vi "sub_removeInvalidGuessFromQueue.vi"() -> ()   [LabVIEW 2018]
uses:
  guess.ctl
panel:
  out "no guesses left ?":bool
  in  "solver (in)":cluster{"solved":bool, "values":string[]}[][](array[cluster]) caption="solver array"
  in  "queues":T1
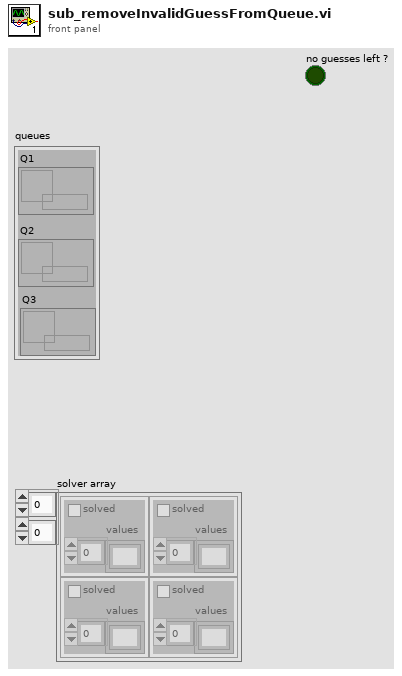
[diagram p1: front panel]
types:
  T1 = cluster{"Q1":refnum<queue>, "Q2":refnum<queue>, "Q3":refnum<queue>}
  T2 = typedef "guess.ctl" = cluster{"cell position":cluster{"row":i32, "col":i32}, "guess":string}
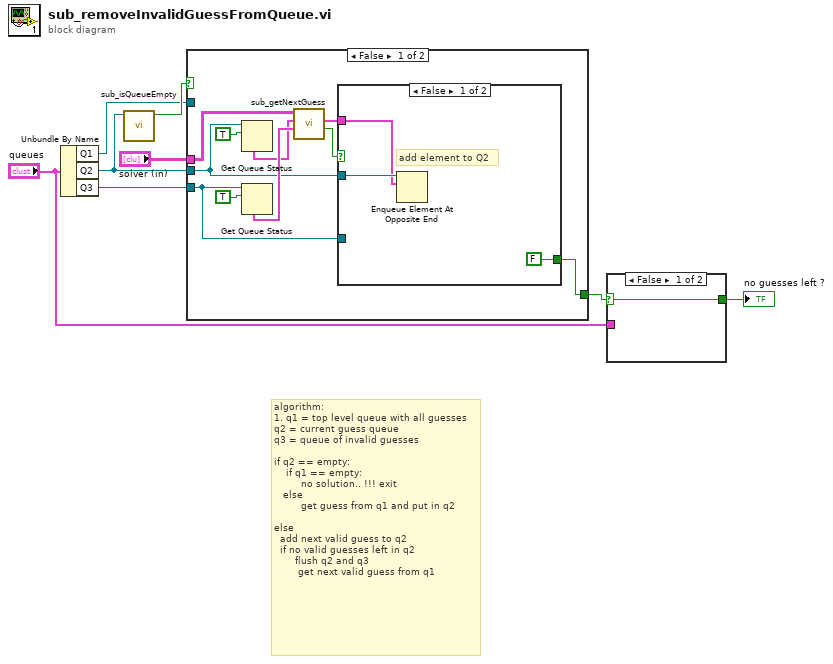
[diagram p0: block diagram]
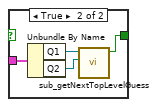
[diagram p2: hidden frame]
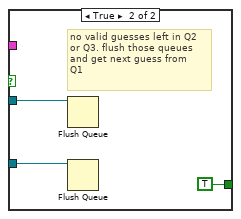
[diagram p3: hidden frame]
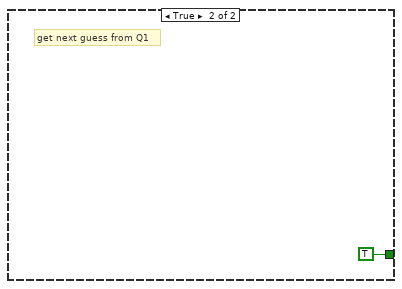
[diagram p4: hidden frame]
diagram:
  # "algorithm:\n1. q1 = top level queue with all guesses\nq2 = current guess queue\nq3 = queue of invalid guesses\n\nif q2 == empty: \n    if q1 == empty: \n         no solution.. !!! exit\n   else\n         get guess from q1 and put in q2\n\nelse\n  add next valid guess to q2\n  if no valid guesses left in q2\n       flush q2 and q3\n        get next valid guess from q1"
  n1 = Unbundle By Name("queues") -> ("Q1"=w7:refnum<queue>, "Q2"=w6:refnum<queue>, "Q3"=w5:refnum<queue>)
  n2 = call "sub_isQueueEmpty"("Q1"=w6) -> ("empty ?"=w8:bool)  [unwired: 10 in]
  n3 = case shown="False" w8 {
    tunnel: w7 -> [_ _]
    tunnel: w6 -> [w12 _]
    tunnel: w5 -> [w11 _]
    tunnel: "solver (in)" -> [w14 _]
    tunnel: [w9 TRUE] -> w3
    frame False {
      n4 = Get Queue Status(queue=w12, return elements? (F)=TRUE) -> (elements=w15:T2[])  [unwired: 1 in, 7 out]
      n5 = Get Queue Status(queue=w11, return elements? (F)=TRUE) -> (elements=w17:T2[])  [unwired: 1 in, 7 out]
      n6 = call "sub_getNextGuess.vi"("invalid guesses"=w17, "current guess queue"=w15, "solver array"=w14) -> ("no valid guess ?"=w13:bool, "next guess"=w10:T2)  [unwired: 7 in]
      n7 = case shown="False" w13 {
        tunnel: w12 -> [w21 w24]
        tunnel: w11 -> [_ w23]
        tunnel: w10 -> [w20 _]
        tunnel: [FALSE TRUE] -> w9
        frame False {
          # "add element to Q2"
          n8 = Enqueue Element At Opposite End(queue=w21, element=w20) -> ()  [unwired: 2 in, 3 out]
        }
        frame True {
          # "no valid guesses left in Q2 \nor Q3. flush those queues\nand get next guess from\nQ1"
          n9 = Flush Queue(queue=w24) -> ()  [unwired: 1 in, 3 out]
          n10 = Flush Queue(queue=w23) -> ()  [unwired: 1 in, 3 out]
        }
      }
    }
    frame True {
      # "get next guess from Q1"
    }
  }
  n11 = case shown="False" w3 {
    selector: w3 -> [w26 _]
    tunnel: "queues" -> [_ w30]
    tunnel: [w26 w27] -> w1
    frame False {
    }
    frame True {
      n12 = Unbundle By Name(w30) -> ("Q1"=w29:refnum<queue>, "Q2"=w28:refnum<queue>)
      n13 = call "sub_getNextTopLevelGuess.vi"("Q2"=w28, "Q1"=w29) -> ("q1 empty ?"=w27:bool)  [unwired: 9 in]
    }
  }
  "no guesses left ?" <- w1
